vi "Method_Const.vi"(4 "Boolean":bool, 5 "A":refnum<class "Abs_Boolean.lvclass">) -> (1 "Result":T1)   [LabVIEW 2021, in "NOR_Bool.lvclass"]
uses:
  NOR_Bool.lvclass
  Abs_Types/Boolean/Abs_Boolean.lvclass
  Abs_Type.ctl
  C:/TSA/LV_Abstract/Source/Functions/Support/Function/Two Terminal/Boolean/AbsFunc_Two Term_Bool.lvclass
  C:/Program Files (x86)/National Instruments/LabVIEW 2021/vi.lib/TSA/Abstract Data Classes/Abs_Types/Boolean/Abs_Boolean.lvclass
  Support/Function/Two Terminal/Boolean/AbsFunc_Two Term_Bool.lvclass/AbsFunc_Two Term_Bool.ctl
  Support/Function/Two Terminal/Boolean/Properties/Write Bool A.vi
  Support/Function/Two Terminal/Boolean/Properties/Write Bool B.vi
  Constants/Support/Bool/Const_Bool.lvclass
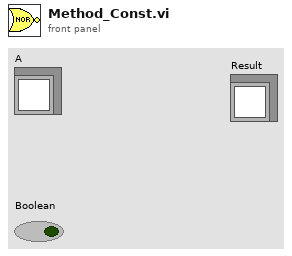
[diagram p1: front panel]
types:
  T1 = typedef "NOR_Bool.lvclass/Abs_Type.ctl" = refnum<class "Abs_Boolean.lvclass">
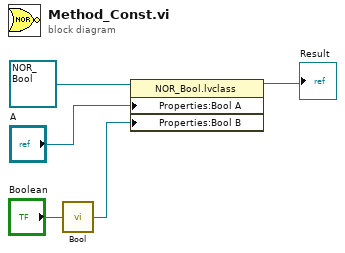
[diagram p0: block diagram]
diagram:
  n1 = call "Bool.vi"("Boolean"="Boolean") -> ("Abs_Boolean.lvclass"=w2:refnum<class "Abs_Boolean.lvclass">)  [unwired: 4 in]
  n2 = property class="NOR_Bool.lvclass"(reference=refnum<class "NOR_Bool.lvclass"> refnum ("Functions.lvlib:Logic.lvlib:AND.lvclass"), "Properties:Bool A"="A", "Properties:Bool B"=w2) -> (reference out=→"Result":refnum<class "NOR_Bool.lvclass">)  [unwired: 1 in, 1 out]
